vi "log_marginal_likelihood.vi"(8 "error in (no error)":errorcluster caption="entrée d'erreur (pas d'erreur)", 11 "GaussianProcessClassifier.lvclass 2":refnum<class "GaussianProcessClassifier.lvclass">) -> (0 "error out":errorcluster caption="sortie d'erreur", 2 "out":T1, 3 "GaussianProcessClassifier.lvclass":refnum<class "GaussianProcessClassifier.lvclass">)   [LabVIEW 2020, in "GaussianProcessClassifier.lvclass"]
doc: "Returns log-marginal likelihood of theta for training data.\n\n In the case of multi-class classification, the mean log-marginal\n likelihood of the one-versus-rest classifiers are returned."
uses:
  GaussianProcessClassifier.lvclass
  C:/Users/cipop/TDF Dropbox/2_Technologies de France/1 - Services et Etudes/PLAIY/2 - DEV/PLAIYLAB/code/Python/Python.lvclass
  C:/Users/cipop/TDF Dropbox/2_Technologies de France/1 - Services et Etudes/PLAIY/2 - DEV/PLAIYLAB/code/Model/Model.lvclass
  GaussianProcessClassifier.lvclass/GaussianProcessClassifier.ctl
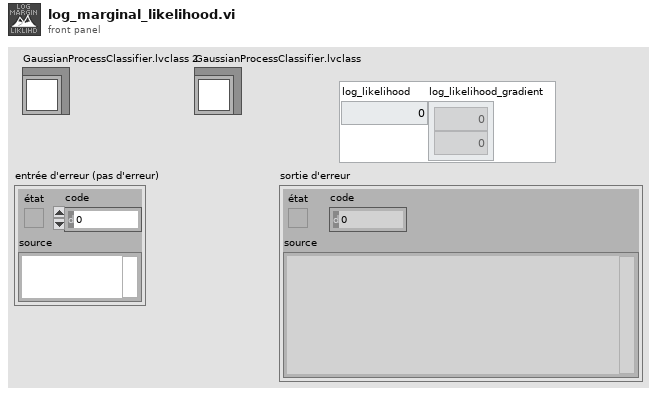
[diagram p1: front panel]
types:
  T1 = cluster{"log_likelihood":dbl, "log_likelihood_gradient":dbl[]}
  T2 = typedef "data.ctl" = cluster{"name":string, "X":dbl[][]}
  T3 = typedef "gaussian_process_classifier_data.ctl" = cluster{"y":dbl[], "sample_weight":dbl[], "clone_kernel":bool}
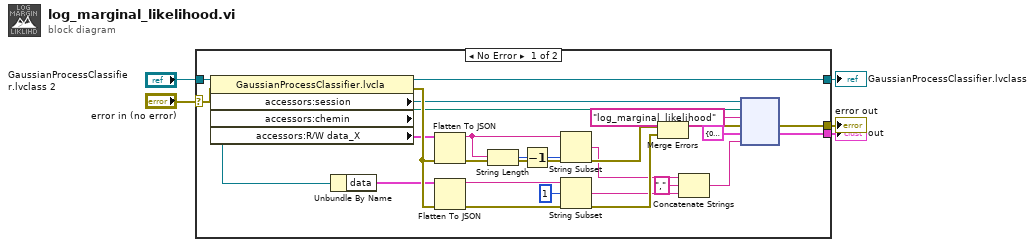
[diagram p0: block diagram]
diagram:
  n1 = case shown="No Error" "error in (no error)" {
    selector: "error in (no error)" -> [w27 w31]
    tunnel: [w28 w31] -> w4
    tunnel: [w10 w30] -> w2
    tunnel: "GaussianProcessClassifier.lvclass 2" -> [w9 w30]
    tunnel: [w7 _] -> w1
    frame No Error {
      n2 = property class="GaussianProcessClassifier.lvcla"(reference=w9, error in=w27) -> (reference out=w10:refnum<class "GaussianProcessClassifier.lvclass">, error out=w23:errorcluster, "accessors:session"=w13:refnum<k35>, "accessors:chemin"=w12:path, "accessors:R/W data_X"=w14:T2)
      n3 = Unbundle By Name(w9) -> ("data"=w8:T3)
      n4 = Flatten To JSON(anything=w14, error in (no error)=w23) -> (JSON string=w24:string, 11:w19:errorcluster)  [unwired: 1 in]
      n5 = Flatten To JSON(anything=w8, error in (no error)=w23) -> (JSON string=w21:string, 11:w20:errorcluster)  [unwired: 1 in]
      n6 = String Length(string=w24) -> (length=w26:i32)
      n7 = Decrement(x=w26) -> (x-1=w25:i32)
      n8 = String Subset(string=w24, length (rest)=w25) -> (substring=w17:string)  [unwired: 1 in]
      n9 = String Subset(string=w21, offset (0)=1) -> (substring=w16:string)  [unwired: 1 in]
      n10 = Merge Errors(w19, w20) -> (w11:errorcluster)
      n11 = Concatenate Strings(w17, "," ("string"), w16) -> (w15:string)
      n12 = node(w13, w12, "log_marginal_likelihood" ("nom de la fonction"), w11, T1 {"log_likelihood"=0.0, "log_likelihood_gradient"=[]} ("out"), w15) -> (w28:errorcluster, w7:T1)  [unwired: 1 in, 3 out]
    }
    frame Error {
    }
  }
  "error out" <- w4
  "GaussianProcessClassifier.lvclass" <- w2
  "out" <- w1
